vi "Bind Terminal Value.vi"(4 "Ignore Past Updates? (F)":bool, 6 "Value Changes Only? (T)":bool=TRUE, 8 "error in (no error)":errorcluster, 9 "Datum Name (\"\"=Use Control Label)":string, 10 "Ctl Refnum":refnum<vi>, 11 "IViewable in":refnum<class "IViewable.lvclass">) -> (0 "error out":errorcluster, 3 "IViewable out":refnum<class "IViewable.lvclass">)   [LabVIEW 2017, in "IViewable.lvlib" / "IViewable.lvclass"]
doc: "Bind the value of a control terminal (control or indicator) to a publication."
uses:
  IViewable.lvclass
  C:/Program Files (x86)/National Instruments/LabVIEW 2017/vi.lib/ActorFramework/Actor/Actor.lvclass
  <vilib>/ActorFramework/Actor/Actor.lvclass/Actor.ctl
  <vilib>/ActorFramework/Message Enqueuer/Message Enqueuer.lvclass/Message Enqueuer.ctl
  SubscriptionPolicy/BasicSubscription/BasicSubscription.lvclass/BasicSubscription.ctl
  SubscriptionPolicy/ValueChangeSubscription/ValueChangeSubscription.lvclass/ValueChangeSubscription.ctl
  IMediator/SubscriptionRequest/SubscriptionRequest.lvclass/SubscriptionRequest.ctl
  IObserver/IObserver Messages/Subscribe Msg/Subscribe Msg.lvclass/Subscribe Msg.ctl
  <vilib>/ActorFramework/Message Enqueuer/Init from Existing Queue.vi
  <vilib>/ActorFramework/Message Enqueuer/Enqueue.vi
  SubscriptionPolicy/BasicSubscription/BasicSubscription.lvclass
  C:/Git/mva-framework/Framework/IMediator/ISubscriptionPolicy/ISubscriptionPolicy.lvclass
  SubscriptionPolicy/ValueChangeSubscription/ValueChangeSubscription.lvclass
  Transport/TerminalBinding/TerminalBinding.lvclass
  C:/Git/mva-framework/Framework/IMediator/ITransport/ITransport.lvclass
  IObserver/IObserver Messages/Subscribe Msg/Subscribe Msg.lvclass
  C:/Program Files (x86)/National Instruments/LabVIEW 2017/vi.lib/ActorFramework/Message/Message.lvclass
  <vilib>/ActorFramework/Message Priority Queue/Priority Enqueue.vi
  <vilib>/ActorFramework/Message Enqueuer/Message Enqueuer.lvclass
  IMediator/SubscriptionRequest/SubscriptionRequest.lvclass
  <vilib>/ActorFramework/Actor/Actor.lvclass
  IMediator/ISubscriptionPolicy/ISubscriptionPolicy.lvclass
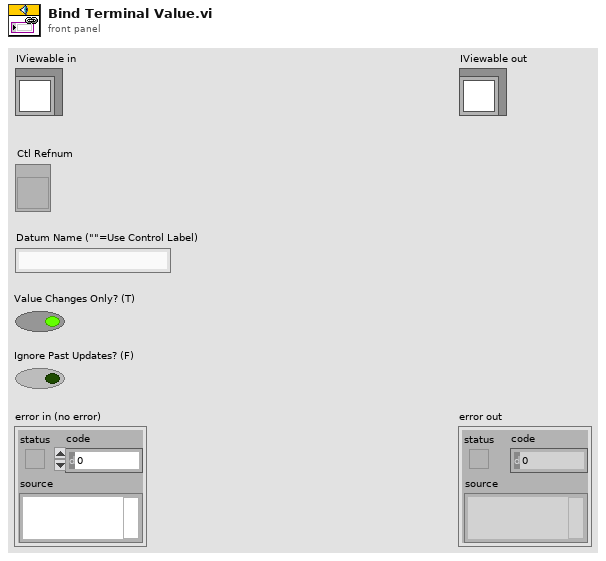
[diagram p1: front panel]
types:
  T1 = typedef "IMediator.lvlib/ISubscriptionPolicy.lvclass/ISubscriptionPolicy Reference.ctl" = refnum<data-value>
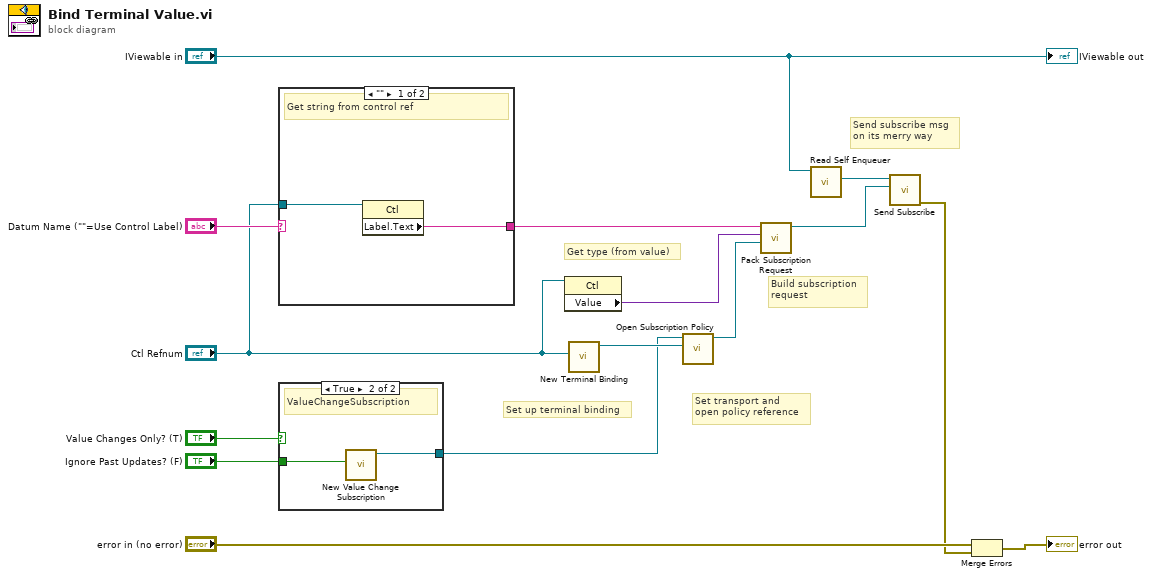
[diagram p0: block diagram]
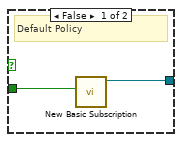
[diagram p2: hidden frame]
diagram:
  # "Set transport and\nopen policy reference"
  # "Send subscribe msg\non its merry way"
  # "Build subscription\nrequest"
  # "Get type (from value)"
  # "Set up terminal binding"
  n1 = case shown="\"\"" "Datum Name (\"\"=Use Control Label)" {
    selector: "Datum Name (\"\"=Use Control Label)" -> [_ w18]
    tunnel: [w16 w18] -> w7
    tunnel: "Ctl Refnum" -> [w17 _]
    frame "" {
      # "Get string from control ref"
      n2 = property class="Ctl"(reference=w17) -> ("Label.Text"=w16:string)  [unwired: 1 in, 2 out]
    }
    frame Default {
      # "Use string wired to input terminal"
    }
  }
  n3 = case shown="True" "Value Changes Only? (T)" {
    tunnel: "Ignore Past Updates? (F)" -> [w19 w22]
    tunnel: [w20 w21] -> w3
    frame False {
      # "Default Policy"
      n4 = call "New Basic Subscription.vi"("Ignore Past Updates? (F)"=w19) -> ("BasicSubscription Out"=w20:refnum<class "BasicSubscription.lvclass">)  [unwired: 10 in]
    }
    frame True {
      # "ValueChangeSubscription"
      n5 = call "New Value Change Subscription.vi"("Ignore Past Updates? (F)"=w22) -> ("ValueChangeSubscription Out"=w21:refnum<class "ValueChangeSubscription.lvclass">)  [unwired: 10 in]
    }
  }
  n6 = property class="Ctl"(reference="Ctl Refnum") -> ("Value"=w14:variant)  [unwired: 1 in, 2 out]
  n7 = call "New Terminal Binding.vi"("Ctl Refnum"="Ctl Refnum") -> ("TerminalBinding"=w5:refnum<class "TerminalBinding.lvclass">)  [unwired: 9 in, 1 out]
  n8 = call "Open Subscription Policy.vi"("Transport"=w5, "SubscriptionPolicy"=w3) -> ("Subscription Policy"=w1:T1)  [unwired: 8 in, 1 out]
  n9 = call "Pack Subscription Request.vi"("Subscription Policy"=w1, "Type"=w14, "Datum Name"=w7) -> ("SubscriptionRequest"=w11:refnum<class "SubscriptionRequest.lvclass">)  [unwired: 8 in]
  n10 = call <vilib>:"Read Self Enqueuer.vi"("Actor"="IViewable in") -> ("Self Enqueuer"=w12:refnum<class "Message Enqueuer.lvclass">)  [unwired: 10 in]
  n11 = call "Send Subscribe.vi"("SubscriptionRequest"=w11, "Message Enqueuer"=w12) -> ("error out"=w9:errorcluster)  [unwired: 8 in, 1 out]
  n12 = Merge Errors("error in (no error)", w9) -> (→"error out":errorcluster)
  "IViewable out" <- "IViewable in"
